vi "Hello World Gif.vi"() -> ()   [LabVIEW 2015]
panel:
  in  "getSmaller":bool
  in  "Size":dbl
  in  "Blue":dbl(slide) scale=0.0..255.0
  in  "Green":dbl(slide) scale=0.0..255.0
  in  "Red":dbl(slide) scale=0.0..255.0
  out "Hello World!":picture
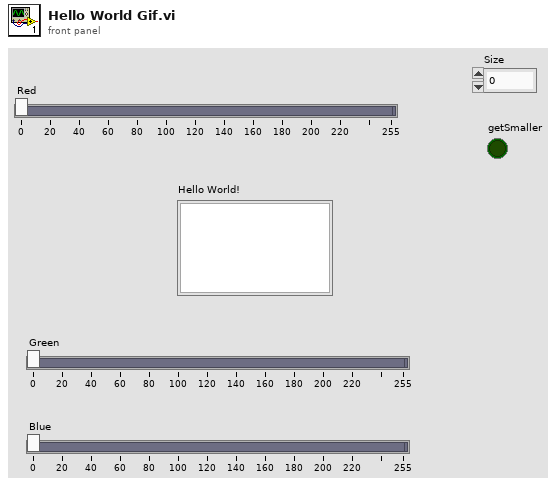
[diagram p1: front panel]
types:
  T1 = cluster{string, "Size":dbl, bool, bool, bool, bool, bool, bool}
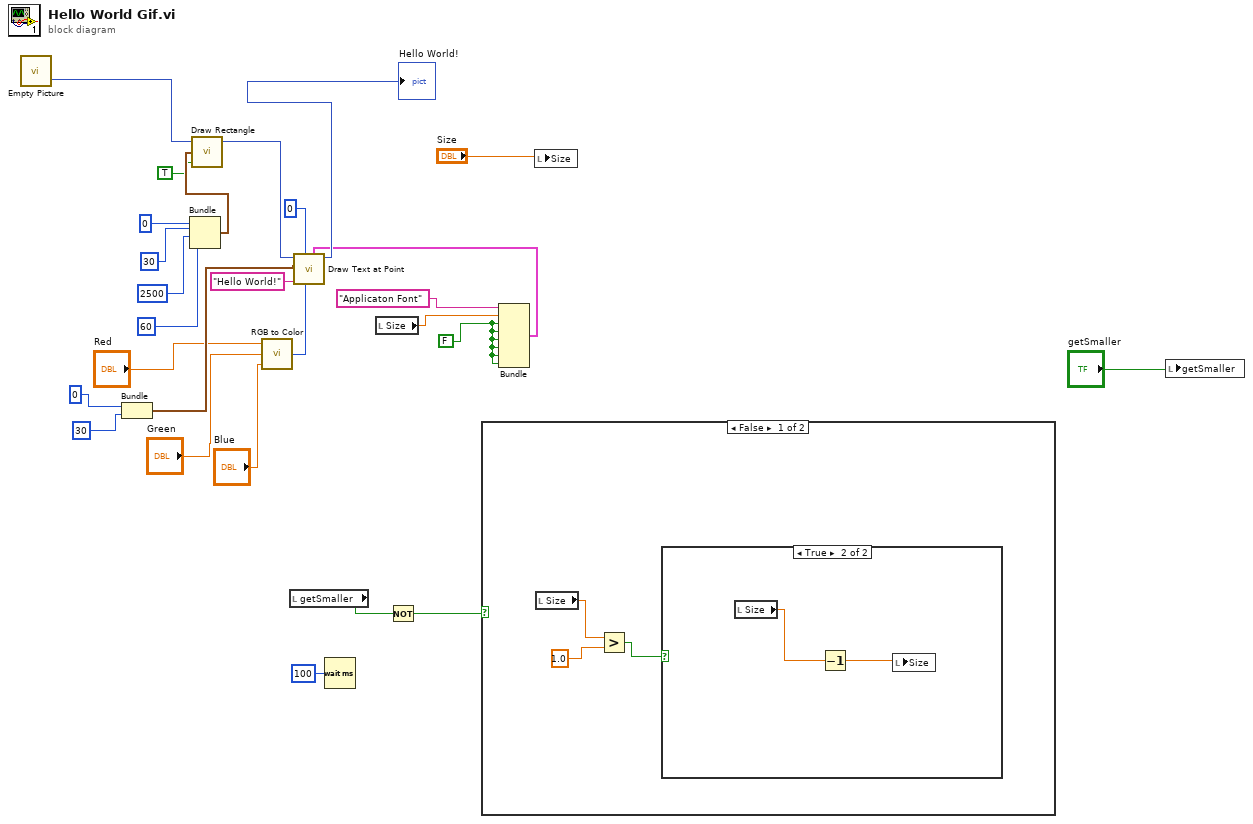
[diagram p0: block diagram]
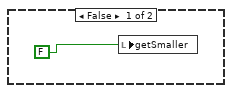
[diagram p2: hidden frame]
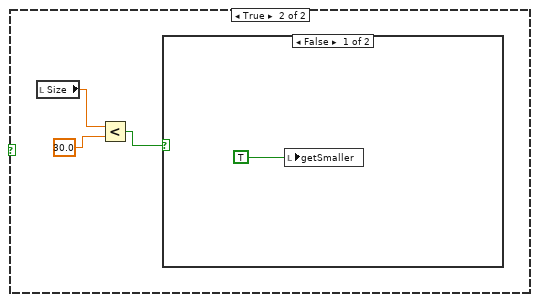
[diagram p3: hidden frame]
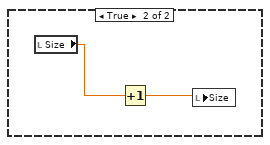
[diagram p4: hidden frame]
diagram:
  w13 = FALSE
  n1 = call "Empty Picture"() -> ("empty picture"=w10:picture)
  n2 = Bundle(i16 0, i16 30) -> (w15:cluster{i16, i16})  [unwired: 1 in]
  n3 = Bundle(0, 30, 2500, 60) -> (w23:cluster{i32, i32, i32, i32})  [unwired: 1 in]
  n4 = call <vilib>:"Draw Rectangle.vi"("picture"=w10, "rect"=w23, "fill?(F)"=TRUE) -> ("new picture"=w21:picture)  [unwired: 6 in]
  n5 = call <vilib>:"RGB to Color.vi"("B"="Blue", "G"="Green", "R"="Red") -> ("Color"=w19:u32)
  n6 = local read "getSmaller"() -> (w1:bool)
  n7 = Wait (ms)(milliseconds to wait=u32 100) -> ()  [unwired: 1 out]
  n8 = local read "Size"() -> (w5:dbl)
  n9 = Not(x=w1) -> (.not. x?=w2:bool)
  n10 = case shown="False" w2 {
    frame False {
      n11 = local read "Size"() -> (w30:dbl)
      n12 = Greater?(x=w30, y=1.0) -> (0:w28:bool)
      n13 = case shown="True" w28 {
        frame False {
          n14 = local write "getSmaller"(FALSE) -> ()
        }
        frame True {
          n15 = local read "Size"() -> (w33:dbl)
          n16 = Decrement(x=w33) -> (x-1=w32:dbl)
          n17 = local write "Size"(w32) -> ()
        }
      }
    }
    frame True {
      n18 = local read "Size"() -> (w36:dbl)
      n19 = Less?(x=w36, y=30.0) -> (x < y?=w34:bool)
      n20 = case shown="False" w34 {
        frame False {
          n21 = local write "getSmaller"(TRUE) -> ()
        }
        frame True {
          n22 = local read "Size"() -> (w39:dbl)
          n23 = Increment(x=w39) -> (x+1=w38:dbl)
          n24 = local write "Size"(w38) -> ()
        }
      }
    }
  }
  n25 = Bundle("Applicaton Font", "Size"=w5, w13, w13, w13, w13, w13, w13) -> (w12:T1)  [unwired: 1 in]
  n26 = call <vilib>:"Draw Text at Point.vi"("[user-specified font]"=w12, "text color(black)"=w19, "desired font(Application)"=0, "text"="Hello World!", "origin"=w15, "picture"=w21) -> ("new picture"=→"Hello World!":picture)  [unwired: 4 in, 1 out]
  n27 = local write "Size"("Size") -> ()
  n28 = local write "getSmaller"("getSmaller") -> ()
